vi "SoundLoop.vi"(8 "error in (no error)":errorcluster, 10 "SoundsFolder":path=path "/home/lvuser/natinst/bin/data/sounds", 11 "Engine in":refnum<class "Engine.lvclass">) -> (0 "error out":errorcluster)   [LabVIEW 2019, in "RT_Game.lvlib" / "Engine.lvclass"]
uses:
  Engine.lvclass
  Engine.lvclass/Engine.ctl
  PlaySoundData.ctl
  ChangeVolumeData.ctl
  <vilib>/Utility/error.llb/Error Cluster From Error Code.vi
  <vilib>/rvi/errors/niLvFpgaAdjustHostInterfaceError.vi
  <vilib>/rvi/interface/common/niFpgaWaitOnOcc.vi
  <vilib>/rvi/interface/nirviReadWriteControl/nirviReadWriteControl.xnode
  FPGA_Interface.ctl
  FPGA Bitfiles/myriogameconsole_FPGATarget_Main_ntsPRcBZGxk.lvbitx
  <vilib>/rvi/interface/nirviMethod/nirviMethod.xnode
  <vilib>/rvi/errors/niLvFpgaMergeErrorWithErrorCode.vi
  NiFpgaLv.dll
  <vilib>/FPGAPlugInAG/myRIO-1900/niLvFpga_ConfigureFifo_myRIO-1900.vi
  <vilib>/FPGAPlugInAG/myRIO-1900/niLvFpga_WriteFifo_myRIO-1900.vi
panel:
  out "Numeric":i32
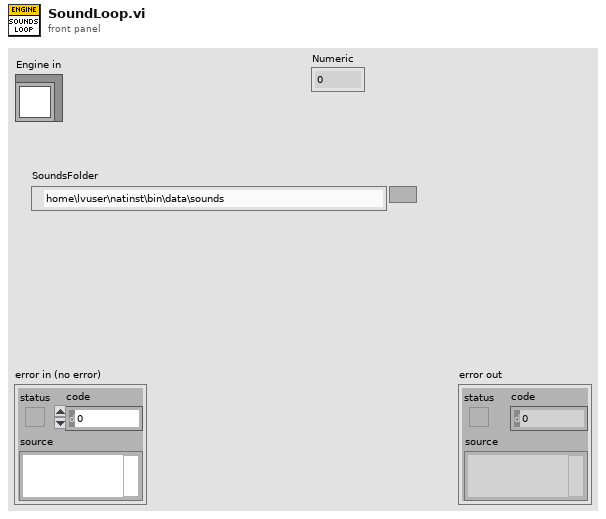
[diagram p1: front panel]
types:
  T1 = typedef "RT_Game.lvlib/Engine.lvclass/PlaySoundData.ctl" = cluster{"Name":string, "Overwrite":bool}
  T2 = typedef "RT_Game.lvlib/Engine.lvclass/ChangeVolumeData.ctl" = enum16{"up", "down", "mute"}
  T3 = typedef "FPGA_Interface.ctl" = refnum<k20>
  T4 = typedef "RT_Game.lvlib/Engine.lvclass/MessageCluster.ctl" = cluster{"Message":string, "Data":variant}
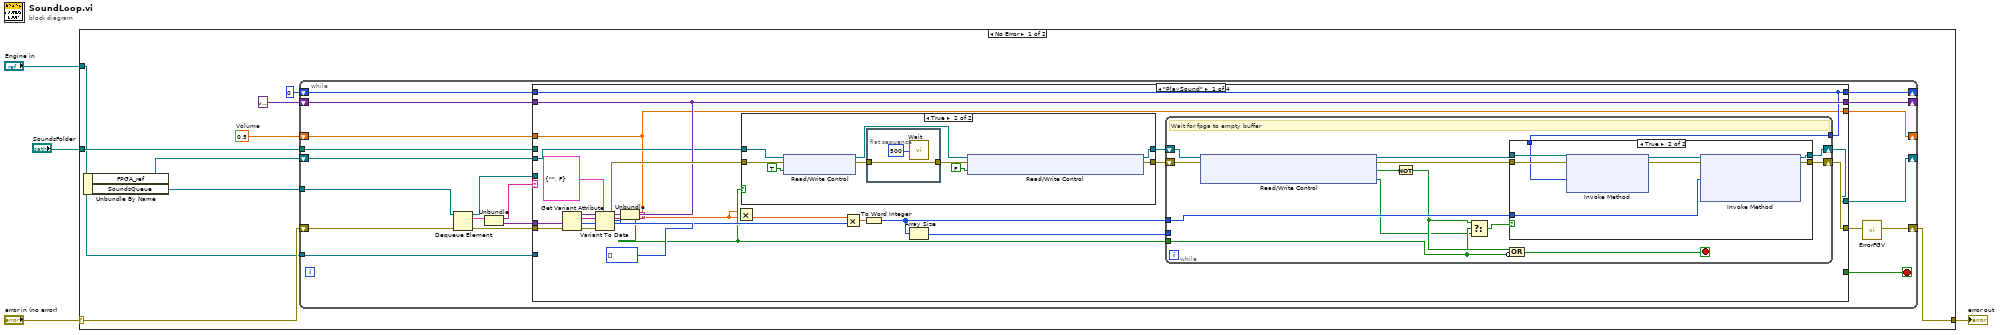
[diagram p0: block diagram]
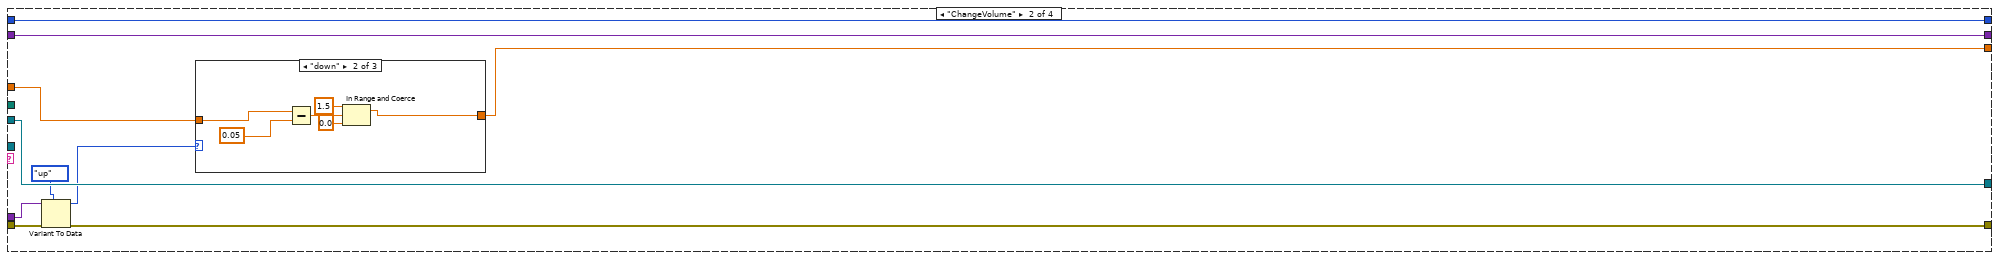
[diagram p4: hidden frame]
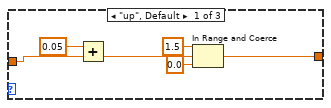
[diagram p5: hidden frame]
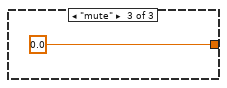
[diagram p6: hidden frame]
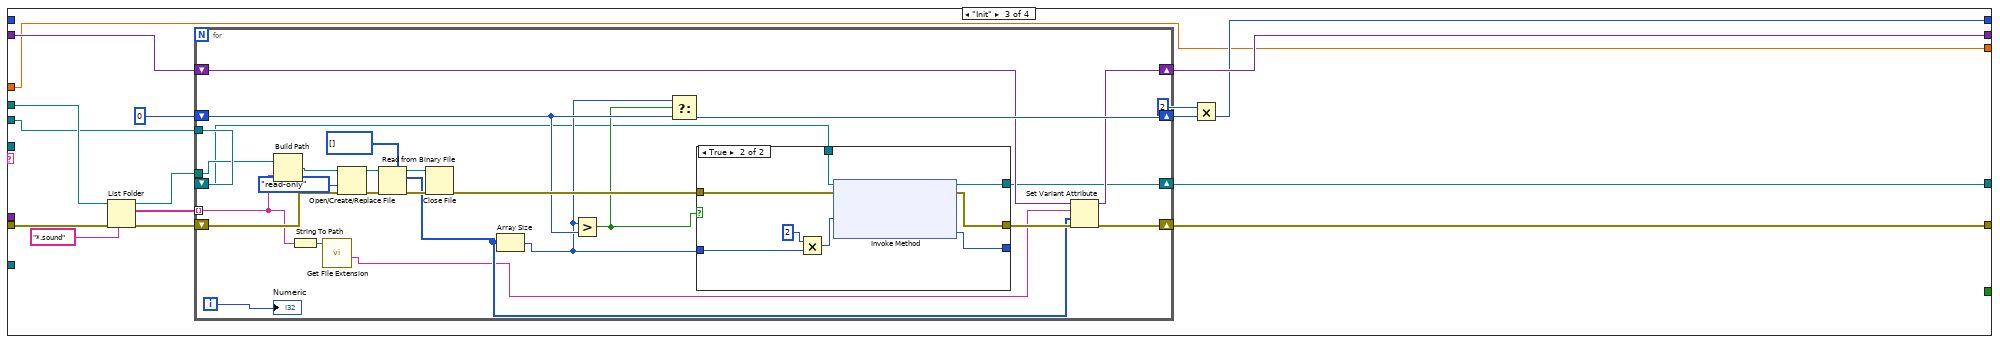
[diagram p7: hidden frame]
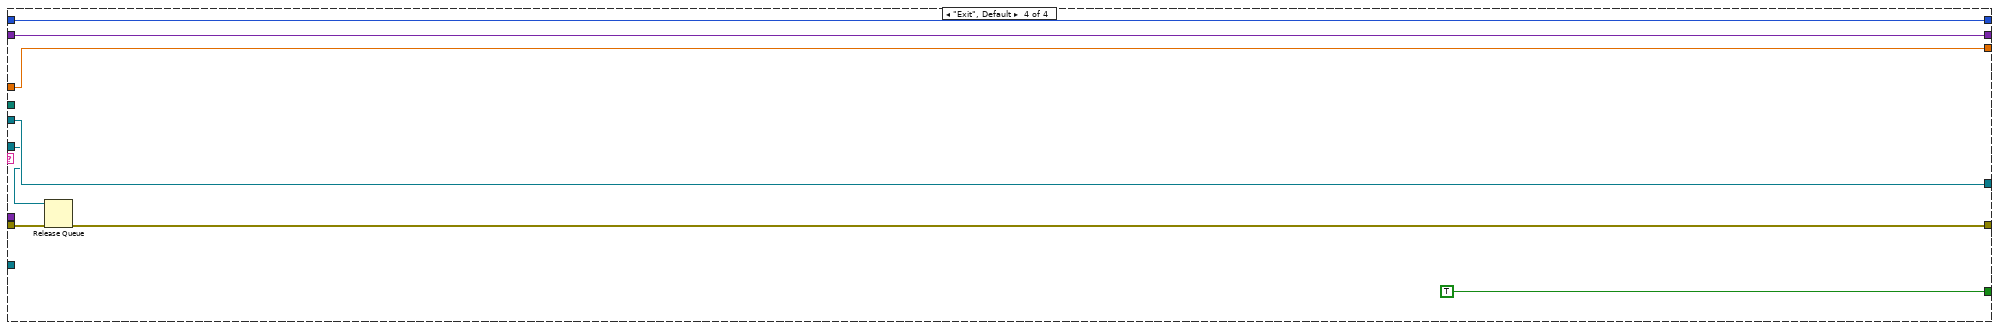
[diagram p9: hidden frame]
diagram:
  n1 = case shown="No Error" "error in (no error)" {
    selector: "error in (no error)" -> [w13 w175]
    tunnel: [w12 w175] -> w3
    tunnel: "Engine in" -> [w9 _]
    tunnel: "SoundsFolder" -> [w10 _]
    frame No Error {
      w6 = 0.5  # Volume
      n2 = Unbundle By Name(w9) -> ("FPGA_ref"=w5:T3, "SoundsQueue"=w11:refnum<queue>)
      n3 = while {
        shift-right: [w15] -> w12
        shift-left: w13 -> [w33]
        tunnel: w11 -> [w31]
        tunnel: w10 -> [w25]
        tunnel: w9 -> [w24]
        shift-right: [w22] -> _
        shift-left: variant -> [w23]
        shift-right: [w20] -> _
        shift-left: w5 -> [w26]
        shift-right: [w19] -> _
        shift-left: 0 -> [w18]
        shift-right: [w16] -> _
        shift-left: w6 -> [w17]
        stop <- w14 stop-if-true
        n4 = Dequeue Element(queue=w31, error in (no error)=w33) -> (queue out=w27:refnum<queue>, element=w30:T4, error out=w32:errorcluster)  [unwired: 1 in, 1 out]
        n5 = Unbundle(w30) -> ("Message"=w29:string, "Data"=w28:variant)
        n6 = case shown="\"PlaySound\"" w29 {
          tunnel: w32 -> [w55 w102 w131 w174]
          tunnel: w28 -> [w47 w96 _ _]
          tunnel: w27 -> [_ _ _ w167]
          tunnel: w26 -> [w37 w100 w120 w171]
          tunnel: w25 -> [_ _ w130 _]
          tunnel: w24 -> [_ _ _ _]
          tunnel: [_ _ _ TRUE] -> w14
          tunnel: [w51 w97 w128 w168] -> w21
          tunnel: w23 -> [w49 w101 w123 w173]
          tunnel: [w49 w101 w124 w173] -> w22
          tunnel: [w38 w100 w121 w171] -> w20
          tunnel: [w36 w99 w118 w170] -> w19
          tunnel: w18 -> [w36 w99 _ w170]
          tunnel: w17 -> [w34 w98 w116 w169]
          tunnel: [w34 w93 w116 w169] -> w16
          frame "PlaySound" {
            n7 = Variant To Data(error in=w55, type=T1 {"Name"="", "Overwrite"=FALSE}, Variant=w47) -> (data=w45:T1, error out=w48:errorcluster)
            n8 = Unbundle(w45) -> ("Name"=w41:string, "Overwrite"=w42:bool)
            n9 = Get Variant Attribute(Variant=w49, name=w41, default value (empty Variant)=i16[] [], error in=w48) -> (value=w43:i16[], error out=w50:errorcluster)  [unwired: 2 out]
            n10 = Multiply(x=w34, y=w34) -> (x*y=w35:dbl)
            n11 = case shown="True" w42 {
              tunnel: w50 -> [w56 w66]
              tunnel: w37 -> [w57 w65]
              tunnel: [w57 w62] -> w52
              tunnel: [w56 w58] -> w53
              frame False {
              }
              frame True {
                n12 = xnode "Read/Write Control"("FPGA VI Reference In"=w65, "error in"=w66, "SoundBuffer_Flush"=TRUE) -> ("FPGA VI Reference Out"=w63:T3, "error out"=w60:errorcluster)
                n13 = flat-sequence {
                  tunnel: [w67] -> w59
                  tunnel: w60 -> [w67]
                  frame #0 {
                    n14 = call "Wait"("Count(uSec)"=u32 500) -> ()  [unwired: 1 out]
                  }
                }
                n15 = xnode "Read/Write Control"("FPGA VI Reference In"=w63, "error in"=w59, "SoundBuffer_Flush"=FALSE) -> ("FPGA VI Reference Out"=w62:T3, "error out"=w58:errorcluster)
              }
            }
            n16 = Multiply(x=w35, y=w43) -> (x*y=w54:dbl[])
            n17 = To Word Integer(number=w54) -> (16bit integer=w40:i16[])
            n18 = Array Size(array=w40) -> (size(s)=w39:i32)
            n19 = while {
              tunnel: w40 -> [w80]
              shift-right: [w81] -> w38
              shift-left: w52 -> [w76]
              shift-right: [w82] -> w51
              shift-left: w53 -> [w79]
              tunnel: w42 -> [w71]
              tunnel: w39 -> [_]
              tunnel: w36 -> [w69]
              stop <- w78 stop-if-true
              # "Wait for fpga to empty buffer"
              n20 = xnode "Read/Write Control"("FPGA VI Reference In"=w76, "error in"=w79) -> ("FPGA VI Reference Out"=w75:T3, "error out"=w77:errorcluster, "SoundBufferFlushing"=w74:bool, "SoundBufferTimeout"=w70:bool)
              n21 = Not(x=w74) -> (.not. x?=w73:bool)
              n22 = Select(t=w73, s=w71, f=w70) -> (s? t:f=w72:bool)
              n23 = case shown="True" w72 {
                tunnel: [w83 w92] -> w82
                tunnel: [w84 w91] -> w81
                tunnel: w80 -> [_ w90]
                tunnel: w75 -> [w84 w87]
                tunnel: w77 -> [w83 w89]
                tunnel: w69 -> [_ w85]
                frame False {
                }
                frame True {
                  n24 = xnode "Invoke Method"("FPGA VI Reference In"=w87, "error in"=w89, "Requested Depth"=w85) -> ("FPGA VI Reference Out"=w86:T3, "error out"=w88:errorcluster)  [unwired: 1 out]
                  n25 = xnode "Invoke Method"("FPGA VI Reference In"=w86, "error in"=w88, "Data"=w90) -> ("FPGA VI Reference Out"=w91:T3, "error out"=w92:errorcluster)  [unwired: 1 in, 1 out]
                }
              }
              n26 = Compound Arithmetic op=OR(w73, invert w71) -> (w78:bool)
            }
          }
          frame "ChangeVolume" {
            n27 = Variant To Data(error in=w102, type=ChangeVolumeData."up", Variant=w96) -> (data=w95:T2, error out=w97:errorcluster)
            n28 = case shown="\"down\"" w95 {
              tunnel: w98 -> [w108 w114 _]
              tunnel: [w105 w109 0.0 ("Volume")] -> w93
              frame "up", Default {
                n29 = Add(x=0.05, y=w108) -> (x+y=w107:dbl)
                n30 = In Range and Coerce(upper limit=1.5, x=w107, lower limit=0.0) -> (coerced(x)=w105:dbl)  [unwired: 1 out]
              }
              frame "down" {
                n31 = Subtract(x=w114, y=0.05 ("x")) -> (x-y=w113:dbl)
                n32 = In Range and Coerce(upper limit=1.5, x=w113, lower limit=0.0) -> (coerced(x)=w109:dbl)  [unwired: 1 out]
              }
              frame "mute" {
              }
            }
          }
          frame "Init" {
            n33 = List Folder(path=w130, pattern="*.sound", error in=w131) -> (path out=w126:path, filenames=w127:string[], error out=w129:errorcluster)  [unwired: 1 in, 1 out]
            n34 = for {
              shift-right: [w143] -> w128
              shift-left: w129 -> [w151]
              tunnel: w127 -> [w139] mode=indexing
              tunnel: w126 -> [w149]
              shift-right: [w146] -> w119
              shift-left: 0 -> [w147]
              tunnel: w120 -> [_]
              shift-right: [w141] -> w124
              shift-left: w123 -> [w142]
              shift-right: [w136] -> w121
              shift-left: w120 -> [w135]
              i -> [w132]
              n35 = Build Path(base path=w149, name or relative path=w139) -> (appended path=w133:path)
              n36 = String To Path(string=w139) -> (path=w138:path)
              n37 = call <vilib>:"Get File Extension.vi"("file"=w138) -> ("filename without extension"=w137:string)  [unwired: 6 in, 4 out]
              n38 = Open/Create/Replace File(file path (use dialog)=w133, error in=w151, access (0:read/write)=enum16{"read/write", "read-only", "write-only"}."read-only") -> (refnum out=w155:refnum<file>, error out=w152:errorcluster)  [unwired: 3 in, 1 out]
              n39 = Read from Binary File(5:i16[] [] ("Sample"), 8:w152, 11:w155) -> (0:w153:errorcluster, 2:w140:i16[], 3:w156:refnum<file>)  [unwired: 3 in, 1 out]
              n40 = Close File(refnum=w156, error in=w153) -> (error out=w154:errorcluster)  [unwired: 1 out]
              n41 = Array Size(array=w140) -> (size(s)=w144:i32)
              n42 = Greater?(x=w144, y=w147) -> (0:w145:bool)
              n43 = Select(t=w144, s=w145, f=w147) -> (s? t:f=w146:i32)
              n44 = case shown="True" w145 {
                tunnel: w154 -> [w158 w164]
                tunnel: [w158 w163] -> w150
                tunnel: w144 -> [_ w162]
                tunnel: w135 -> [w157 w161]
                tunnel: [w157 w160] -> w136
                tunnel: [_ w159] -> _
                frame False {
                }
                frame True {
                  n45 = Multiply(x=2, y=w162) -> (x*y=w165:i32)
                  n46 = xnode "Invoke Method"("FPGA VI Reference In"=w161, "error in"=w164, "Requested Depth"=w165) -> ("FPGA VI Reference Out"=w160:T3, "error out"=w163:errorcluster, "Actual Depth"=w159:u32)
                }
              }
              n47 = Set Variant Attribute(Variant=w142, name=w137, value=w140, error in=w150) -> (Variant out=w141:variant, error out=w143:errorcluster)  [unwired: 1 out]
              "Numeric" <- w132
            }
            n48 = Multiply(x=2, y=w119) -> (x*y=w118:i32)
          }
          frame "Exit", Default {
            n49 = Release Queue(queue=w167, error in (no error)=w174) -> (error out=w168:errorcluster)  [unwired: 1 in, 2 out]
          }
        }
        n50 = call "ErrorFGV.vi"("error in (no error)"=w21) -> ("error out"=w15:errorcluster)  [unwired: 9 in, 1 out]
      }
    }
    frame Error {
    }
  }
  "error out" <- w3
